vi "Load StandardWaveForm from SpreadSheet.vi"(11 "Path":path) -> (3 "StandardWaveforms Array":T1[](array[typedef]) {"Waveform"."Time" format="%.0p"; "Waveform"."amplitude" min=0.0 max=1.0 format="%.2p"})   [LabVIEW 2013]
uses:
  StandardWaveformWithName.ctl
  StandardWaveform.ctl
  <vilib>/Utility/file.llb/Read From Spreadsheet File (string).vi
panel:
  in  "Cluster":T1={"Name"="", "Waveform"={"waveform type"=enum."sine", "amplitude"=1.0, "Time"=256.0}} {"Waveform"."amplitude" min=0.0 max=1.0 format="%.2f"}
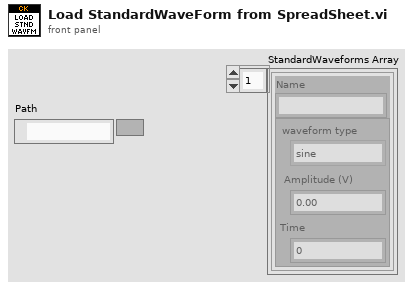
[diagram p1: front panel]
types:
  T1 = typedef "StandardWaveformWithName.ctl" = cluster{"Name":string, "Waveform":T2}
  T2 = typedef "StandardWaveform.ctl" = cluster{"waveform type":enum16{"sine", "cosine", "triangle", "square", "sawtooth", "increasing ramp", "decreasing ramp", "DC Value"}, "amplitude":dbl, "Time":dbl}
  T3 = enum16{"sine", "cosine", "triangle", "square", "sawtooth", "increasing ramp", "decreasing ramp", "DC Value"}
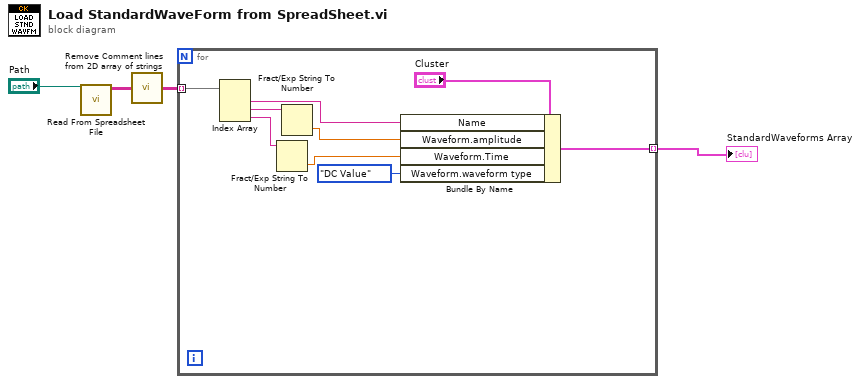
[diagram p0: block diagram]
diagram:
  n1 = call-poly <vilib>:"Read From Spreadsheet File.vi"("file path (dialog if empty)"="Path") -> ("all rows"=w2:string[][])  [unwired: 6 in, 4 out]
  n2 = call "Remove Comment lines from 2D array of strings.vi"("Array in"=w2) -> ("Array out"=w1:string[][])
  n3 = for {
    tunnel: w1 -> [w11] mode=indexing
    tunnel: [w5] -> w4 mode=indexing
    n4 = Index Array(array=w11) -> (element #1=w10:string, element #2=w9:string, element #3=w6:string)  [unwired: 3 in]
    n5 = Fract/Exp String To Number(string=w6) -> (number=w7:dbl)  [unwired: 3 in, 1 out]
    n6 = Fract/Exp String To Number(string=w9) -> (number=w8:dbl)  [unwired: 3 in, 1 out]
    n7 = Bundle By Name(cluster="Cluster", "Name"=w10, "Waveform.amplitude"=w8, "Waveform.Time"=w7, "Waveform.waveform type"=T3."DC Value") -> (w5:T1)
  }
  "StandardWaveforms Array" <- w4
